vi "forward proj comparison.vi"(4 "number of projections":u32, 6 "Angles":dbl[](array[numeric]), 7 "path name":path, 8 "source tiff pointer":i64 format="%x", 9 "Centre":i32[](array[numeric]), 10 "Output":u8[](array[numeric]), 11 "Image Properties":T1) -> ()   [LabVIEW 2013]
uses:
  tags_cluster.ctl
  imagereconstruction/x64/Debug/labviewdll.dll
panel:
  out "all forward projections":u8[](array[numeric])
  out "normalised":u8[](array[numeric])
  out "raw":sgl[](array[numeric])
  out "normalisation":i32[](array[numeric])
  out "Current proj":i32
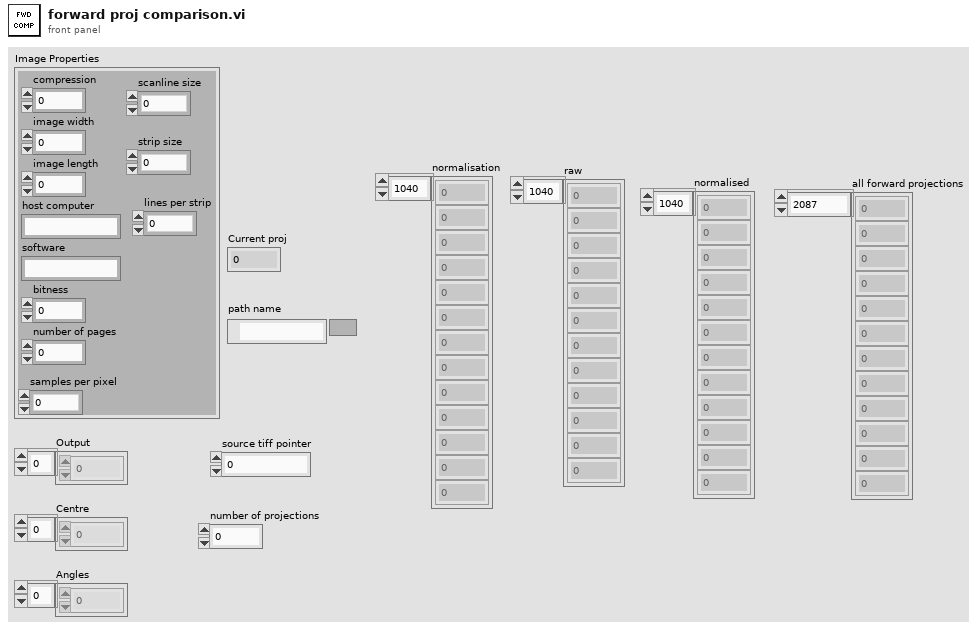
[diagram p1: front panel]
types:
  T1 = typedef "tags_cluster.ctl" = cluster{"compression":i32, "image width":i32, "image length":i32, "host computer":string, "software":string, "bitness":i32, "number of pages":i32, "samples per pixel":i32, "scanline size":i32, "strip size":i32, "lines per strip":i32}
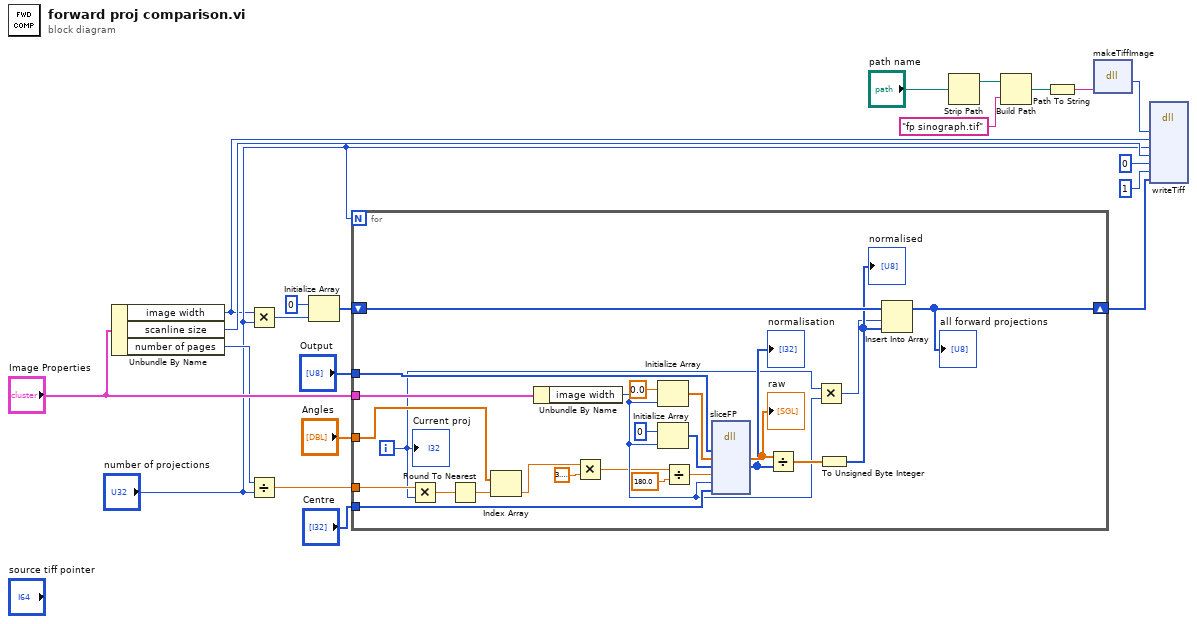
[diagram p0: block diagram]
diagram:
  n1 = Unbundle By Name("Image Properties") -> ("image width"=w1:i32, "scanline size"=w9:i32, "number of pages"=w5:i32)
  n2 = Multiply(x=w1, y="number of projections") -> (x*y=w3:u32)
  n3 = Divide(x=w5, y="number of projections") -> (x/y=w4:dbl)
  n4 = Initialize Array(u8 0 ("element"), w3) -> (w13:u8[])
  n5 = for {
    N: "number of projections" -> [_]
    tunnel: "Output" -> [w46]
    tunnel: "Image Properties" -> [w45]
    tunnel: "Angles" -> [w34]
    tunnel: "Centre" -> [w44]
    shift-right: [w35] -> w6
    shift-left: w13 -> [w37]
    tunnel: w4 -> [w33]
    i -> [w29]
    n6 = Multiply(x=w33, y=w29) -> (x*y=w32:dbl)
    n7 = Round To Nearest(number=w32) -> (nearest integer value=w31:dbl)
    n8 = Index Array(array=w34, index=w31) -> (element=w26:dbl)
    n9 = Unbundle By Name(w45) -> ("image width"=w27:i32)
    n10 = Multiply(x=w26, y=3.141592653589793) -> (x*y=w25:dbl)
    n11 = Initialize Array(sgl 0.0 ("element"), w27) -> (w42:sgl[])
    n12 = Initialize Array(0 ("element"), w27) -> (w40:i32[])
    n13 = Divide(x=w25, y=180.0) -> (x/y=w22:dbl)
    n14 = dll-call lib="D:/work/uni/FYP/reconrepo/imagereconstruction/x64/Debug/labviewdll.dll" fn="sliceFP"("object"=w46, "projection"=w42, "normalisation"=w40, "angle"=w22, "w"=w27, "centre"=w44) -> ("projection"=w39:sgl[], "normalisation"=w38:i32[])  [unwired: 8 in, 2 out]
    "normalisation" <- w38
    "raw" <- w39
    n15 = Divide(x=w39, y=w38) -> (x/y=w36:sgl[])
    n16 = Multiply(x=w29, y=w27) -> (x*y=w28:i32)
    n17 = To Unsigned Byte Integer(number=w36) -> (unsigned 8bit integer=w30:u8[])
    "normalised" <- w30
    n18 = Insert Into Array(array=w37, index=w28, new element=w30) -> (w35:u8[])
    "all forward projections" <- w35
    "Current proj" <- w29
  }
  n19 = Strip Path(path="path name") -> (stripped path=w17:path)  [unwired: 1 out]
  n20 = Build Path(base path=w17, name or relative path="fp sinograph.tif") -> (appended path=w16:path)
  n21 = Path To String(path=w16) -> (string=w19:string)
  n22 = dll-call lib="D:/work/uni/FYP/reconrepo/imagereconstruction/x64/Debug/labviewdll.dll" fn="makeTiffImage"("pathname"=w19) -> ("return type"=w12:i64)  [unwired: 4 in, 2 out]
  n23 = dll-call lib="D:/work/uni/FYP/reconrepo/imagereconstruction/x64/Debug/labviewdll.dll" fn="writeTiff"("tiff"=w12, "w"=w1, "l"="number of projections", "scanline size"=w9, "page"=0, "npages"=1, "data"=w6) -> ()  [unwired: 11 in, 2 out]
